vi "move2.vi"(4 "error in (no error)":errorcluster, 6 "dst dir":path, 7 "full file path":path) -> (0 "error out":errorcluster)   [LabVIEW 2010]
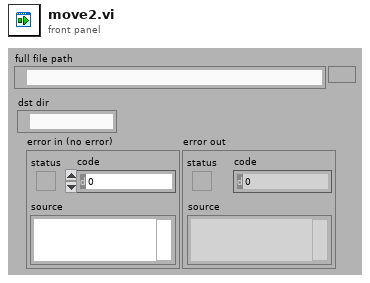
[diagram p1: front panel]
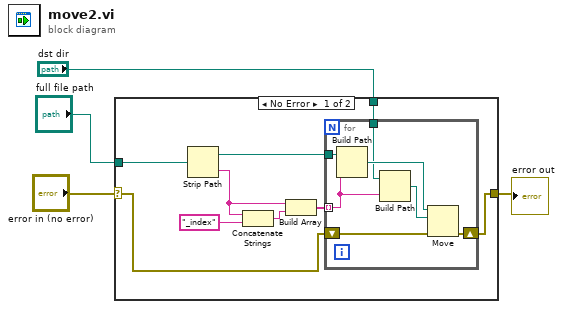
[diagram p0: block diagram]
diagram:
  n1 = case shown="No Error" "error in (no error)" {
    selector: "error in (no error)" -> [w10 w21]
    tunnel: [w9 w21] -> w4
    tunnel: "full file path" -> [w7 _]
    tunnel: "dst dir" -> [w8 _]
    frame No Error {
      n2 = Strip Path(path=w7) -> (stripped path=w5:path, name=w6:string)
      n3 = Concatenate Strings(w6, "_index" ("string")) -> (w12:string)
      n4 = Build Array(w6, w12) -> (w11:string[])
      n5 = for {
        tunnel: w11 -> [w14] mode=indexing
        tunnel: w5 -> [w20]
        shift-right: [w18] -> w9
        shift-left: w10 -> [w19]
        tunnel: w8 -> [w15]
        n6 = Build Path(base path=w20, name or relative path=w14) -> (appended path=w17:path)
        n7 = Build Path(base path=w15, name or relative path=w14) -> (appended path=w16:path)
        n8 = Move(source path=w17, error in=w19, 10:w16) -> (error out=w18:errorcluster)  [unwired: 2 in, 2 out]
      }
    }
    frame Error {
    }
  }
  "error out" <- w4
